vi "EX 10-1 xbee LED test.vi"() -> ()   [LabVIEW 2010]
uses:
  <vilib>/LabVIEW Interface for Arduino/Type Defs/Pin Mode.ctl
  <vilib>/LabVIEW Interface for Arduino/Type Defs/Board Type.ctl
  <vilib>/LabVIEW Interface for Arduino/Type Defs/Connection Type.ctl
  <vilib>/LabVIEW Interface for Arduino/LabVIEW Interface for Arduino.lvlib
panel:
  out ".not. x?":bool
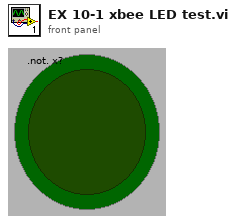
[diagram p1: front panel]
types:
  T1 = typedef "LabVIEW Interface for Arduino.lvlib/Connection Type.ctl" = enum8{"USB / Serial", "XBEE", "BlueSmirf (Bluetooth)"}
  T2 = typedef "LabVIEW Interface for Arduino.lvlib/Board Type.ctl" = enum16{"Uno", "Dimuelanove w/Atmega 328", "Mega 2560"}
  T3 = typedef "LabVIEW Interface for Arduino.lvlib/Pin Mode.ctl" = enum8{"Input", "Output"}
  T4 = typedef "LabVIEW Interface for Arduino.lvlib/Arduino Resource.ctl" = cluster{"VISA resource":refnum<visa-resource-name>, "Board Type":T2, "Connection Type":enum8{"USB / Serial"}, "Bytes Per Packet (15)":u8}
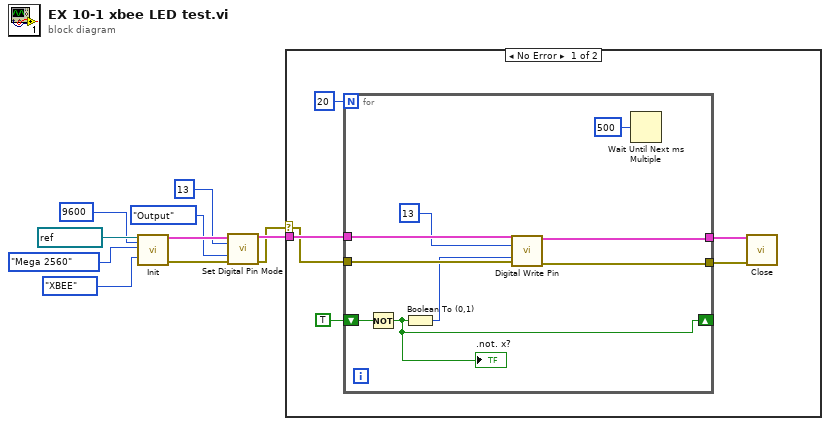
[diagram p0: block diagram]
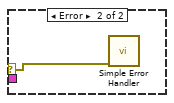
[diagram p2: hidden frame]
diagram:
  n1 = call <vilib>:"Init.vi"("VISA resource"=refnum<visa-resource-name> "COM8", "Baud Rate (115200)"=u32 9600, "Board Type (Uno)"=Board_Type."Mega 2560", "Connection Type (USB/Serial)"=Connection_Type."XBEE") -> ("Arduino Resource"=w10:T4, "error out"=w9:errorcluster)  [unwired: 14 in]
  n2 = call <vilib>:"Set Digital Pin Mode.vi"("Arduino Resource"=w10, "Digital I/O Pin"=u8 13, "Pin Mode (Input)"=Pin_Mode."Output", "error in"=w9) -> ("Arduino Resource"=w4:T4, "error out"=w1:errorcluster)  [unwired: 10 in]
  n3 = case shown="No Error" w1 {
    selector: w1 -> [w11 w26]
    tunnel: w4 -> [w16 _]
    frame No Error {
      n4 = for {
        N: 20 -> [_]
        tunnel: w16 -> [w25]
        tunnel: w11 -> [w24]
        shift-right: [w18] -> _
        shift-left: TRUE -> [w22]
        tunnel: [w20] -> w12
        tunnel: [w19] -> w13
        n5 = Not(x=w22) -> (.not. x?=w18:bool)
        ".not. x?" <- w18
        n6 = Boolean To (0,1)(Boolean=w18) -> (0, 1=w21:i16)
        n7 = call <vilib>:"Digital Write Pin.vi"("Arduino Resource"=w25, "Digital I/O Pin (0)"=u8 13, "Value (0)"=w21, "error in"=w24) -> ("Arduino Resource"=w19:T4, "error out"=w20:errorcluster)  [unwired: 10 in]
        n8 = Wait Until Next ms Multiple(millisecond multiple=u32 500) -> ()  [unwired: 1 out]
      }
      n9 = call <vilib>:"Close.vi"("Arduino Resource"=w13, "error in"=w12) -> ()  [unwired: 13 in, 1 out]
    }
    frame Error {
      n10 = call <vilib>:"Simple Error Handler.vi"("error in (no error)"=w26) -> ()  [unwired: 4 in, 5 out]
    }
  }
